vi "Load Config.vi"(8 "error in (no error)":errorcluster, 11 "Sequencing Control in":refnum<class "Sequencing Control.lvclass">) -> (0 "error out":errorcluster, 3 "Sequencing Control out":refnum<class "Sequencing Control.lvclass">)   [LabVIEW 2020, in "VolatusSeqGUI.lvlib" / "Sequencing Control.lvclass"]
uses:
  Sequencing Control.lvclass
  Sequencing Control.lvclass/Sequencing Control.ctl
  Volatus/VolatusAPI/VolatusAPI.lvclass
  VolatusConfig/VolatusConfigElement/VolatusConfigElement.lvclass
  lv-cdm/CDM-Config/Config Element/Config Element.lvclass
  VolatusConfig/Node/Node Config.lvclass
  C:/dev/lv20CE/relink/lv-volatus/VolatusConfig/VolatusConfigElement/VolatusConfigElement.lvclass
  C:/dev/lv20CE/relink/lv-volatus/VolatusConfig/Node/Node Config.lvclass
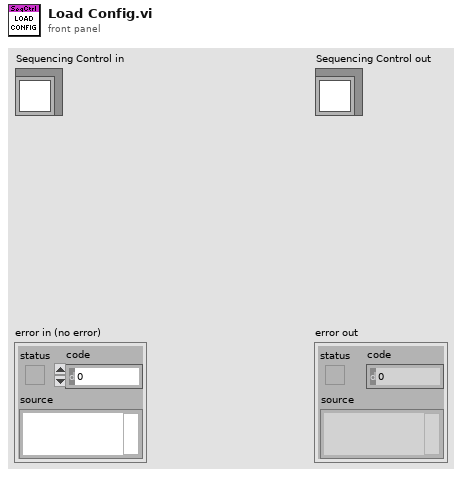
[diagram p1: front panel]
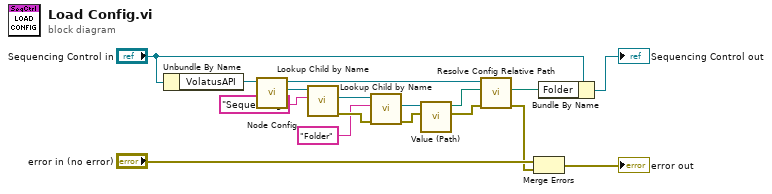
[diagram p0: block diagram]
diagram:
  n1 = Unbundle By Name("Sequencing Control in") -> ("VolatusAPI"=w14:refnum<class "VolatusAPI.lvclass">)
  n2 = call "Node Config.vi"("VolatusAPI in"=w14) -> ("Node Config"=w13:refnum<class "Node Config.lvclass">, "VolatusAPI out"=w9:refnum<class "VolatusAPI.lvclass">)  [unwired: 9 in]
  n3 = call "Lookup Child by Name.vi"("Child Name"="Sequencing", "VolatusConfigElement in"=w13) -> ("error out"=w17:errorcluster, "Child"=w11:refnum<class "Config Element.lvclass">)  [unwired: 6 in, 2 out]
  n4 = call "Lookup Child by Name.vi"("error in (no error)"=w17, "Name"="Folder" ("Child Name"), "Config Element in"=w11) -> ("error out"=w6:errorcluster, "Child"=w8:refnum<class "Config Element.lvclass">)  [unwired: 5 in, 2 out]
  n5 = call "Value (Path).vi"("error in (no error)"=w6, "Config Element in"=w8) -> ("error out"=w5:errorcluster, "Path Value"=w7:path)  [unwired: 8 in]
  n6 = call "Resolve Config Relative Path.vi"("error in (no error)"=w5, "Path"=w7, "VolatusAPI in"=w9) -> ("error out"=w1:errorcluster, "Resolved Path"=w3:path)  [unwired: 6 in, 1 out]
  n7 = Merge Errors("error in (no error)", w1) -> (→"error out":errorcluster)
  n8 = Bundle By Name(cluster="Sequencing Control in", "Folder"=w3) -> (→"Sequencing Control out":refnum<class "Sequencing Control.lvclass">)
